vi "Create Events.vi"(8 "error in (no error)":errorcluster) -> (0 "error out":errorcluster, 2 "Event Regs":refnum<event-registration>, 3 "Events":T1)   [LabVIEW 2017, in "CLI.lvclass"]
uses:
  CLI.lvclass
  CLI.lvclass/CLI.ctl
  Events.ctl
panel:
  # "Connector Pane"
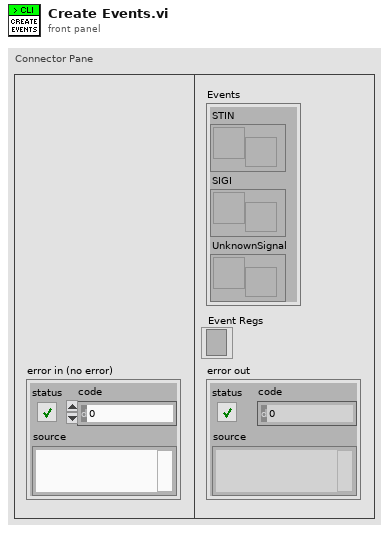
[diagram p1: front panel]
types:
  T1 = typedef "Events.ctl" = cluster{"STIN":refnum<user-event>, "SIGI":refnum<user-event>, "UnknownSignal":refnum<user-event>}
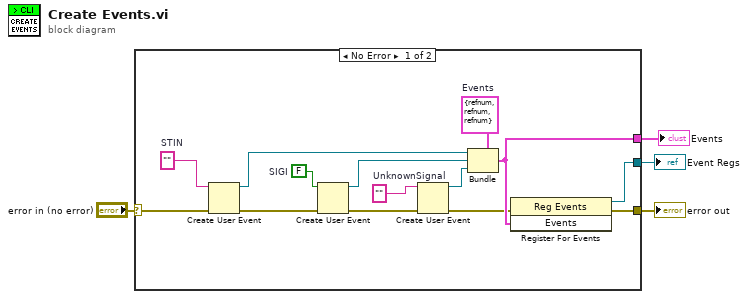
[diagram p0: block diagram]
diagram:
  n1 = case shown="No Error" "error in (no error)" {
    selector: "error in (no error)" -> [w14 w19]
    tunnel: [w15 _] -> w4
    tunnel: [w13 w19] -> w2
    tunnel: [w5 _] -> w1
    frame No Error {
      w9 = ""  # UnknownSignal
      w16 = T1 {"STIN"=refnum, "SIGI"=refnum, "UnknownSignal"=refnum}  # Events
      w18 = FALSE  # SIGI
      w17 = ""  # STIN
      n2 = Create User Event(user event datatype=w17, error in=w14) -> (user event=w11:refnum<user-event>, error out=w12:errorcluster)
      n3 = Create User Event(user event datatype=w18, error in=w12) -> (user event=w10:refnum<user-event>, error out=w8:errorcluster)
      n4 = Create User Event(user event datatype=w9, error in=w8) -> (user event=w6:refnum<user-event>, error out=w7:errorcluster)
      n5 = Bundle(cluster=w16, "STIN"=w11, "SIGI"=w10, "UnknownSignal"=w6) -> (w15:T1)
      n6 = register-events(error in=w7, w15) -> (reference out=w5:refnum<event-registration>, error out=w13:errorcluster)  [unwired: 1 in]
    }
    frame Error {
    }
  }
  "Events" <- w4
  "Event Regs" <- w1
  "error out" <- w2
